vi "GCSArray_header_file.vi"(0 "GCS Array Filepath":path, 5 "error in (no error)":errorcluster, 6 "Block index":i32 min=0 max=0) -> (14 "GCSArray Header":T1={"Identifier"="", "Version"=0, "Remark"="", "Dimension"=0, "Type"=enum."Matrix", "Separator"=0, "NData"=0, "NData%"=[], "Name%"=[], "Start%"=[], "End%"=[], "Delta%"=[], "SampleTime"=inf, "TransmittedUnit%"=[], "DisplayedUnit%"=[], "RatioNominator%"=[], "RatioDenominator%"=[]}, 19 "error out":errorcluster)   [LabVIEW 2026]
doc: "Load specified GCSArray header from file."
uses:
  GCSArray_header.ctl
  GCSArray_regex_selector.ctl
  GCSArray_regex_range.ctl
panel:
  # "Load specified GCSArray header from file."
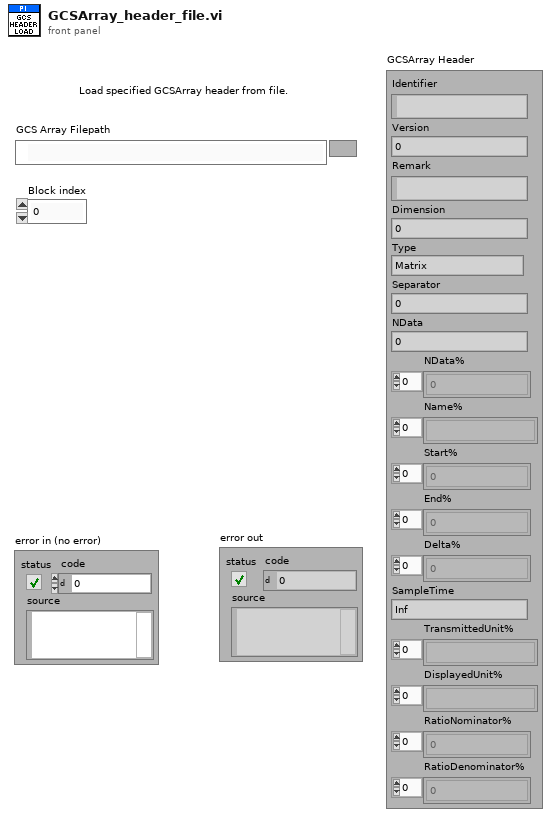
[diagram p1: front panel]
types:
  T1 = typedef "GCSArray_header.ctl" = cluster{"Identifier":string, "Version":i32, "Remark":string, "Dimension":i32, "Type":enum16{"Matrix", "Table"}, "Separator":u8, "NData":i32, "NData%":i32[], "Name%":string[], "Start%":dbl[], "End%":dbl[], "Delta%":dbl[], "SampleTime":dbl, "TransmittedUnit%":string[], "DisplayedUnit%":string[], "RatioNominator%":dbl[], "RatioDenominator%":dbl[]}
  T2 = typedef "GCSArray_regex_range.ctl" = cluster{"Begin":i32, "End":i32}
  T3 = typedef "GCSArray_regex_selector.ctl" = enum16{"GCS_ARRAY Block Full", "GCS_ARRAY Block ID", "GCS_ARRAY Block Header", "GCS_ARRAY Block Data", "GCS_ARRAY Identifier", "GCS_ARRAY Remark", "GCS_ARRAY Version", "GCS_ARRAY Dimension", "GCS_ARRAY Type", "GCS_ARRAY Separator", "GCS_ARRAY NData", "GCS_ARRAY NData%", "GCS_ARRAY NData% Keyword", "GCS_ARRAY Name%", "GCS_ARRAY Name% Keyword", "GCS_ARRAY Start%", "GCS_ARRAY Start% Keyword", "GCS_ARRAY End%", "GCS_ARRAY End% Keyword", "GCS_ARRAY Delta%", "GCS_ARRAY Delta% Keword", "GCS_ARRAY Sample Time", "GCS_ARRAY Unit of transmitted value%", "GCS_ARRAY Trans_Unit% Keyword", "GCS_ARRAY Trans_Unit% = RAW Keyword", "GCS_ARRAY Unit of displayed value%", "GCS_ARRAY Disp_Unit% Keyword", "GCS_ARRAY Nominator%", "GCS_ARRAY Ratio_Nom% Keyword", "GCS_ARRAY Denominator%", "GCS_ARRAY Ratio_Denom% Keyword", "GCS_ARRAY End of Header", "GCS_ARRAY Empty line of Header"}
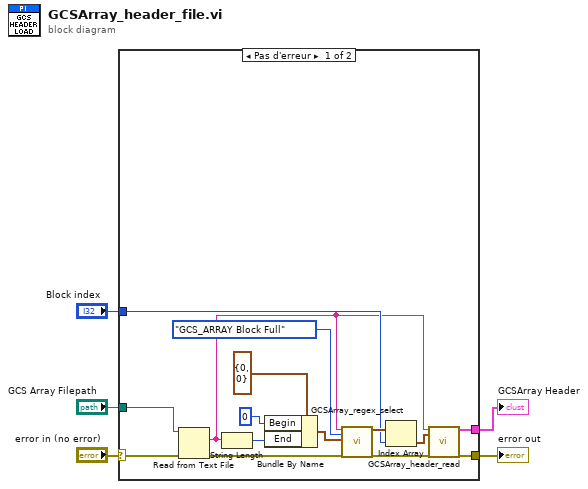
[diagram p0: block diagram]
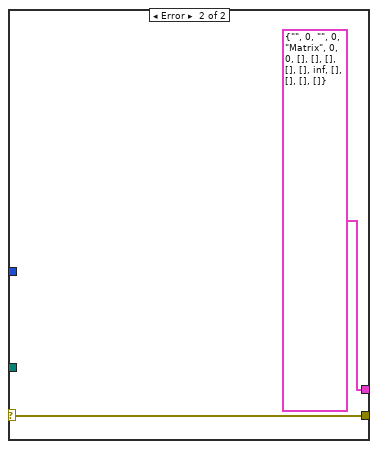
[diagram p2: hidden frame]
diagram:
  n1 = case shown="Pas d'erreur" "error in (no error)" {
    selector: "error in (no error)" -> [w13 w22]
    tunnel: [w9 w22] -> w4
    tunnel: "GCS Array Filepath" -> [w12 _]
    tunnel: "Block index" -> [w11 _]
    tunnel: [w8 T1 {"Identifier"="", "Version"=0, "Remark"="", "Dimension"=0, "Type"=enum."Matrix", "Separator"=0, "NData"=0, "NData%"=[], "Name%"=[], "Start%"=[], "End%"=[], "Delta%"=[], "SampleTime"=inf, "TransmittedUnit%"=[], "DisplayedUnit%"=[], "RatioNominator%"=[], "RatioDenominator%"=[]} ("GCSArray Header")] -> w1
    frame No Error {
      n2 = Read from Text File(file (use dialog)=w12, error in=w13) -> (text=w6:string, error out=w18:errorcluster)  [unwired: 4 out]
      n3 = String Length(string=w6) -> (length=w17:i32)
      n4 = Bundle By Name(cluster=T2 {"Begin"=0, "End"=0} ("Selection"), "Begin"=0, "End"=w17) -> (w20:T2)
      n5 = call "GCSArray_regex_select.vi"("GCSArray input string"=w6, "Selector"=GCSArray_regex_selector."GCS_ARRAY Block Full", "Range"=w20, "error in (no error)"=w18) -> ("Matches"=w19:T2[], "error out"=w10:errorcluster)  [unwired: 14 out]
      n6 = Index Array(array=w19, index=w11) -> (element=w7:T2)
      n7 = call "GCSArray_header_read.vi"("GCSArray input string"=w6, "Range"=w7, "error in (no error)"=w10) -> ("GCSArray Header"=w8:T1, "error out"=w9:errorcluster)  [unwired: 15 in]
    }
    frame Error {
    }
  }
  "error out" <- w4
  "GCSArray Header" <- w1
